vi "LV SciSDK INIT REGISTER FILE.vi"(9 "handle":T2, 10 "Register file name":string) -> (1 "Register File Handle Out":T1)   [LabVIEW 2021]
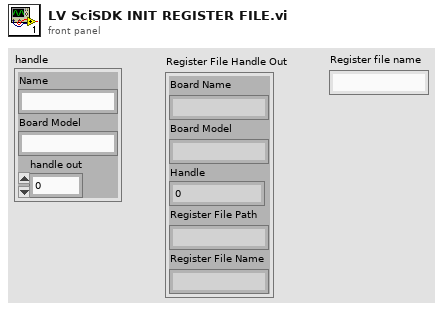
[diagram p1: front panel]
types:
  T1 = cluster{"Board Name":string, "Board Model":string, "Handle":u64, "Register File Path":string, "Register File Name":string}
  T2 = cluster{"Name":string, "Board Model":string, "handle out":u64}
  T3 = cluster{"Name":string, "Board Model":string, "handle out":u64, string, "Register file name":string}
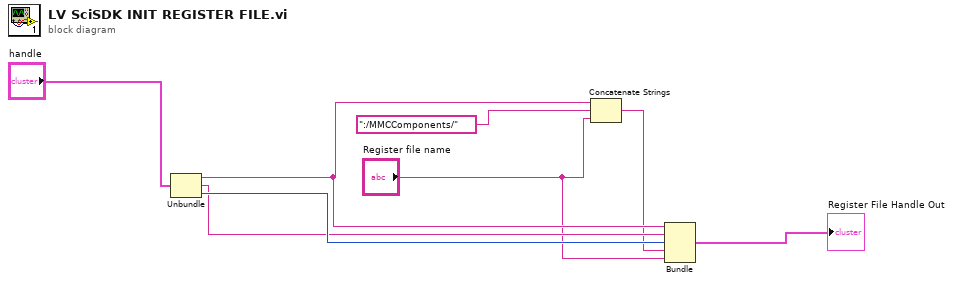
[diagram p0: block diagram]
diagram:
  n1 = Unbundle("handle") -> ("Name"=w5:string, "Board Model"=w3:string, "handle out"=w4:u64)
  n2 = Concatenate Strings(w5, ":/MMCComponents/" ("string"), "Register file name") -> (w2:string)
  n3 = Bundle("Name"=w5, "Board Model"=w3, "handle out"=w4, w2, "Register file name"="Register file name") -> (→"Register File Handle Out":T3)  [unwired: 1 in]
